vi "Large integer U8 array - ADD.vi"(3 "Large number - U8 2":T1, 5 "Large number - U8 1":T1) -> (1 "Added array":T1)   [LabVIEW 2013]
doc: "Adds two large numbers (U8 array format)."
uses:
  User Access Type defs/Large number - U8 array.ctl
panel:
  # "index 0 = LSD"
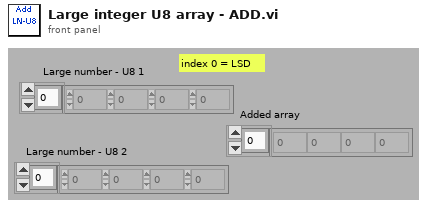
[diagram p1: front panel]
types:
  T1 = typedef "Large number - U8 array.ctl" = u8[]
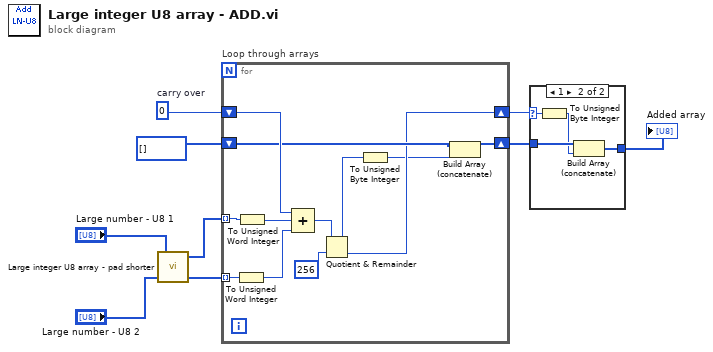
[diagram p0: block diagram]
diagram:
  w4 = u16 0  # carry over
  n1 = call "Large integer U8 array - pad shorter.vi"("Large number -U8 2"="Large number - U8 2", "Large number -U8 1"="Large number - U8 1") -> ("Large number -U8 2 out"=w6:T1, "Large number -U8 1 out"=w7:T1)  [unwired: 2 out]
  n2 = for "Loop through arrays" {
    shift-right: [w19] -> w2
    shift-left: u8[] [] ("Multiplied array") -> [w20]
    shift-right: [w12] -> w3
    shift-left: w4 -> [w21]
    tunnel: w7 -> [w18] mode=indexing
    tunnel: w6 -> [w17] mode=indexing
    n3 = To Unsigned Word Integer(number=w17) -> (unsigned 16bit integer=w15:u16)
    n4 = To Unsigned Word Integer(number=w18) -> (unsigned 16bit integer=w16:u16)
    n5 = Compound Arithmetic op=ADD(w21, w16, w15) -> (w14:u16)
    n6 = Quotient & Remainder(x=w14, y=u16 256) -> (x-y*floor(x/y)=w11:u16, floor(x/y)=w12:u16)
    n7 = To Unsigned Byte Integer(number=w11) -> (unsigned 8bit integer=w10:u8)
    n8 = Build Array (concatenate)(w20, w10) -> (w19:u8[])
  }
  n9 = case shown="1" w3 {
    selector: w3 -> [_ w24]
    tunnel: w2 -> [w22 w26]
    tunnel: [w22 w25] -> w1
    frame 0, Default {
    }
    frame 1 {
      n10 = To Unsigned Byte Integer(number=w24) -> (unsigned 8bit integer=w23:u8)
      n11 = Build Array (concatenate)(w26, w23) -> (w25:u8[])
    }
  }
  "Added array" <- w1
